vi "Load Device Image.vi"(8 "Error In":errorcluster, 10 "Device Type":u16(ring) items=["chipKIT Uno32", "chipKIT uC32", "chipKIT Max32", "chipKIT DP32"], 11 "Device Family":u16(ring) items=["National Instruments", "Digilent", "Arduino"]) -> (0 "Error Out":errorcluster, 1 "Image Found?":bool, 3 "Device Image":picture)   [LabVIEW 2013, in "LVH-LINX.lvlib"]
doc: "Load LINX Device Image"
uses:
  <vilib>/LabVIEW Hacker/LINX/LVH-LINX.lvlib
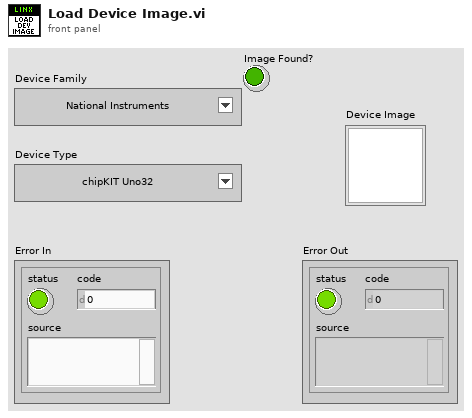
[diagram p1: front panel]
types:
  T1 = typedef "imagedata.ctl" = cluster{"image type":i32, "image depth":i32, "image":u8[], "mask":u8[], "colors":u32[], "Rectangle":cluster{"left":i16, "top":i16, "right":i16, "bottom":i16}}
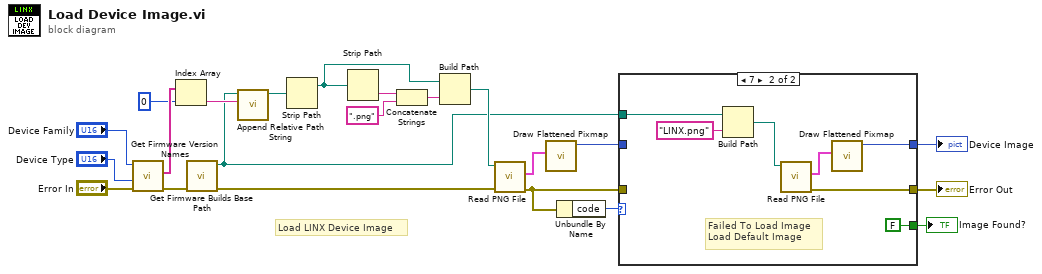
[diagram p0: block diagram]
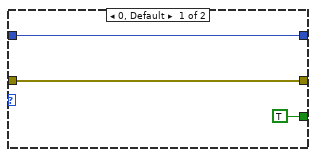
[diagram p2: hidden frame]
diagram:
  # "Load LINX Device Image"
  n1 = call <vilib>:"Get Firmware Version Names.vi"("Error In"="Error In", "Device ID"="Device Type", "Device Family"="Device Family") -> ("Error Out"=w21:errorcluster, "Firmware Version Relative Path"=w22:string[])  [unwired: 6 in, 1 out]
  n2 = Index Array(array=w22, index=0) -> (element=w20:string)
  n3 = call <vilib>:"Get Firmware Builds Base Path.vi"("Error In"=w21) -> ("Error Out"=w9:errorcluster, "Firmware Builds Base Path"=w2:path)  [unwired: 9 in]
  n4 = call <vilib>:"Append Relative Path String.vi"("Relative Path"=w20, "Base Path"=w2) -> ("Absolute Path"=w15:path)  [unwired: 8 in, 1 out]
  n5 = Strip Path(path=w15) -> (stripped path=w12:path)  [unwired: 1 out]
  n6 = Strip Path(path=w12) -> (name=w14:string)  [unwired: 1 out]
  n7 = Concatenate Strings(w14, ".png" ("string")) -> (w11:string)
  n8 = Build Path(base path=w12, name or relative path=w11) -> (appended path=w10:path)
  n9 = call <vilib>:"Read PNG File.vi"("error in (no error)"=w9, "path to PNG file"=w10) -> ("error out"=w6:errorcluster, "image data"=w8:T1)  [unwired: 7 in, 1 out]
  n10 = call <vilib>:"Draw Flattened Pixmap.vi"("image data"=w8) -> ("new picture"=w3:picture)  [unwired: 8 in]
  n11 = Unbundle By Name(w6) -> ("code"=w7:i32)
  n12 = case shown="7" w7 {
    tunnel: w6 -> [w24 _]
    tunnel: [w24 w28] -> w5
    tunnel: [w25 w29] -> w4
    tunnel: w3 -> [w25 _]
    tunnel: w2 -> [_ w32]
    tunnel: [TRUE FALSE] -> w1
    frame 0, Default {
    }
    frame 7 {
      # "Failed To Load Image\nLoad Default Image"
      n13 = Build Path(base path=w32, name or relative path="LINX.png") -> (appended path=w27:path)
      n14 = call <vilib>:"Read PNG File.vi"("path to PNG file"=w27) -> ("error out"=w28:errorcluster, "image data"=w31:T1)  [unwired: 8 in, 1 out]
      n15 = call <vilib>:"Draw Flattened Pixmap.vi"("image data"=w31) -> ("new picture"=w29:picture)  [unwired: 8 in]
    }
  }
  "Error Out" <- w5
  "Device Image" <- w4
  "Image Found?" <- w1
